vi "LEP_RV_ASW_BuildReportTab.vi"() -> ()   [LabVIEW 2011]
uses:
  resource/dialog/PreferencesDialog/optionsFrame_EventData1.ctl
panel:
  out "status display":string="Unknown"
  in  "eval mode?":bool
  in  "path to map file":path
  out "Unused":u32(colorbox)=16777215
  out "Other RAM":u32(colorbox)=12566942
  out "Heap RAM":u32(colorbox)=9328754
  out "RAM (kB)":cluster{dbl, dbl}(slide)={8.35820895522388, 30.80597014925373} scale=0.0..32.0
  out "Flash (kB)":dbl(slide)=29.611940298507463 scale=0.0..64.0
  out "Total Memory (%)":cluster{dbl, dbl, dbl, dbl}(slide)={31.343283582089555, 43.28358208955224, 61.194029850746276, 78.35820895522389} scale=0.0..100.0
  out "Flash Memory":u32(colorbox)=6654652
  out "Unavailable in Evaluation Mode":u32(colorbox)=1381653
  in  "page sync rendezvous":T1
  in  "error msg format string":string="There was a problem applying the options from the %s category. The error message is \"%s.\""
  in  "error in (no error)":errorcluster
  in  "Close Event":refnum<user-event>
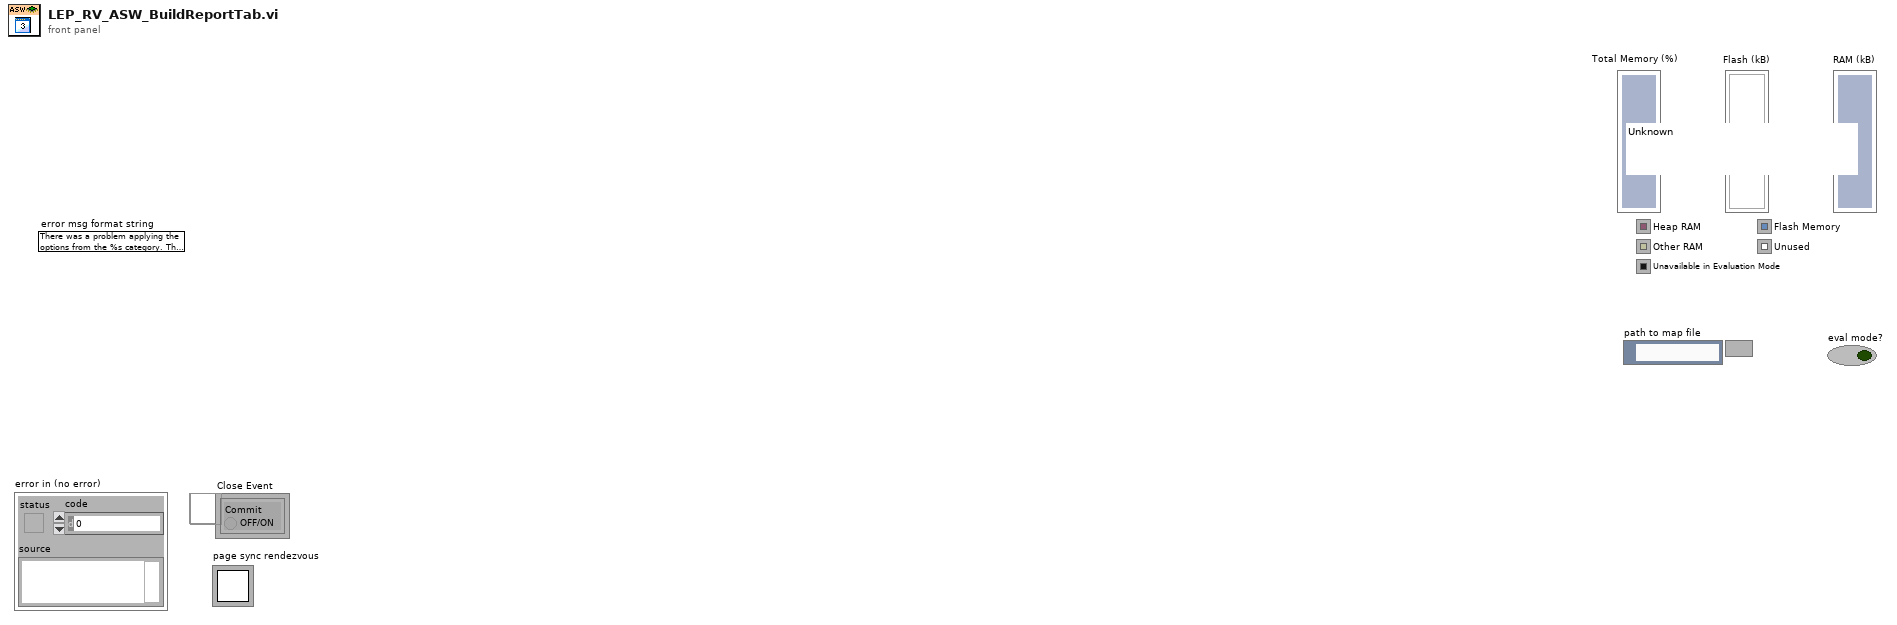
[diagram p1: front panel]
types:
  T1 = typedef "Rendezvous RefNum" = refnum<k1>
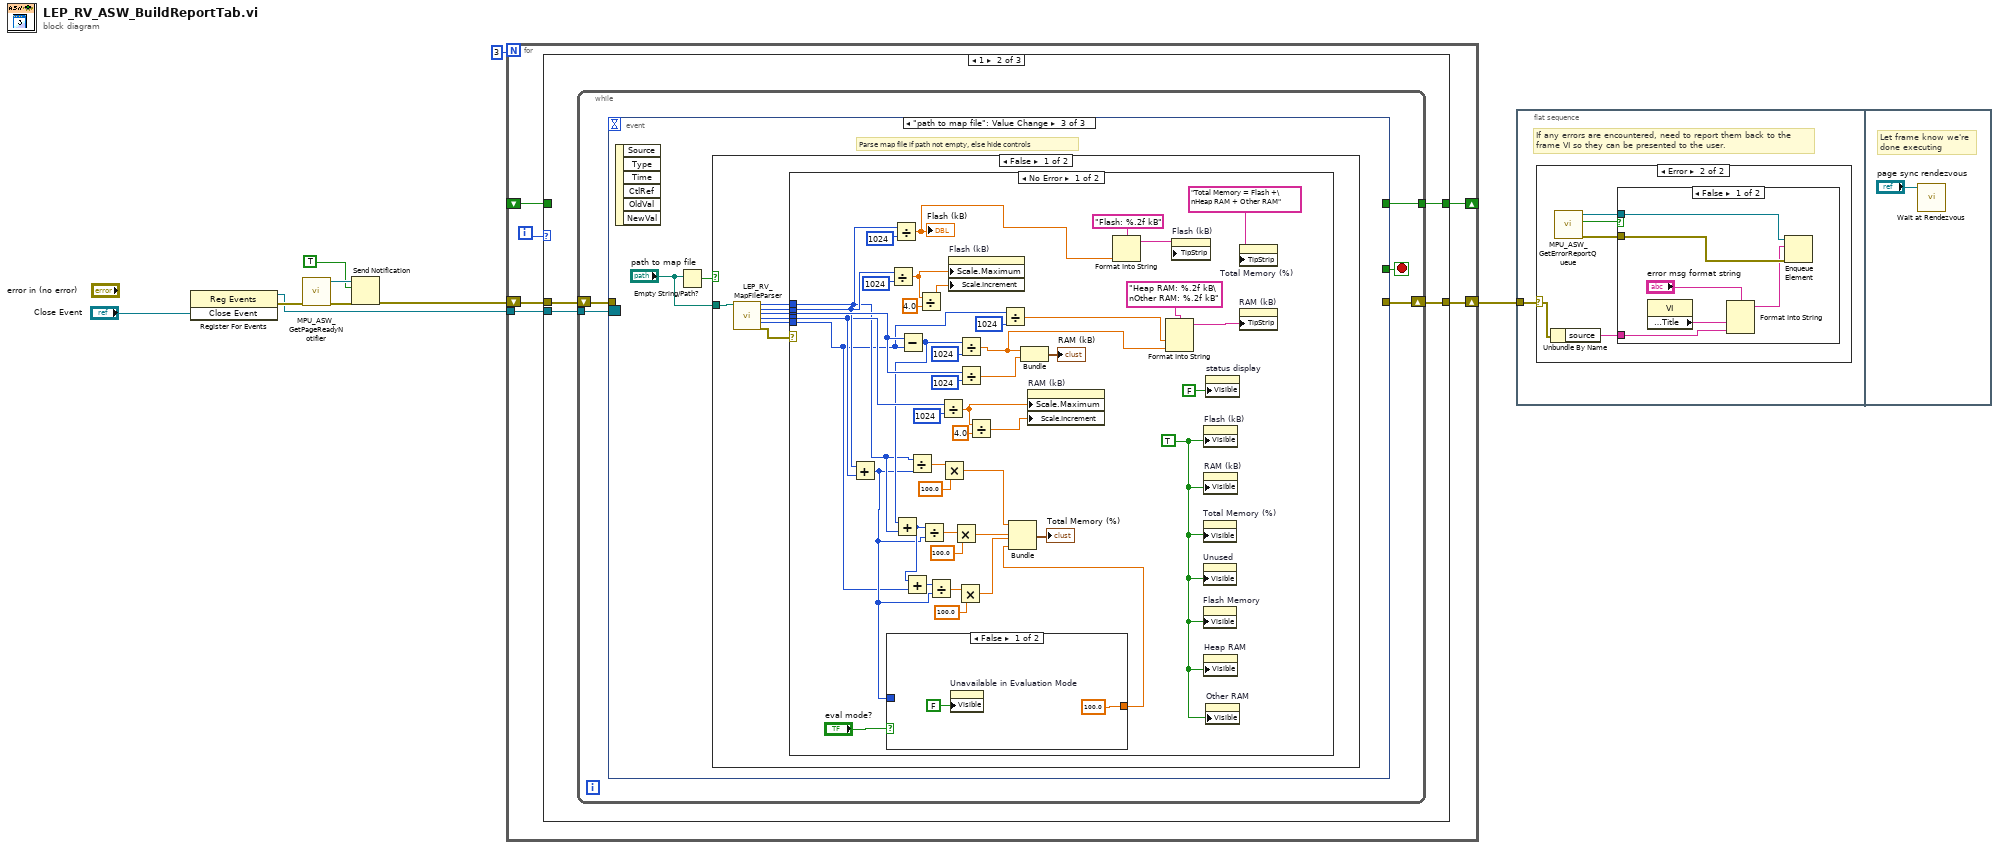
[diagram p0: block diagram]
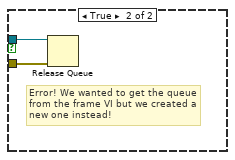
[diagram p3: hidden frame]
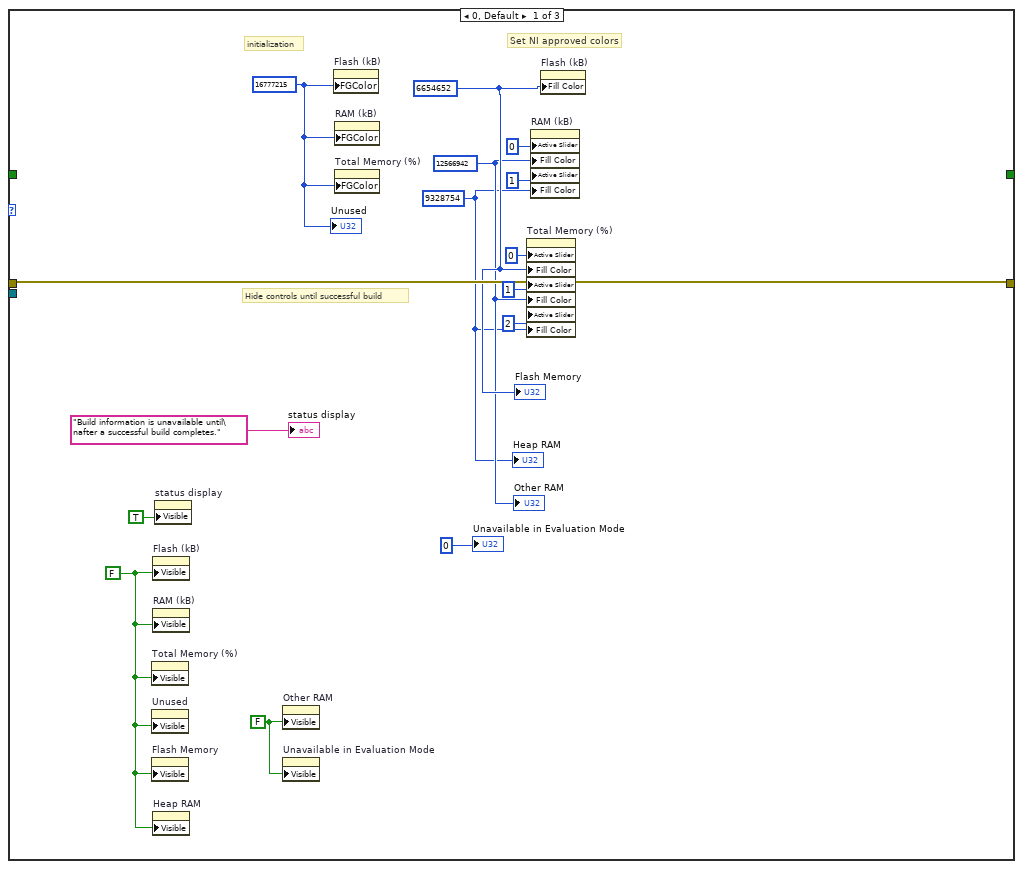
[diagram p4: hidden frame]
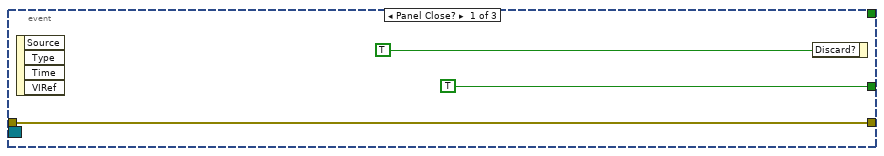
[diagram p5: hidden frame]
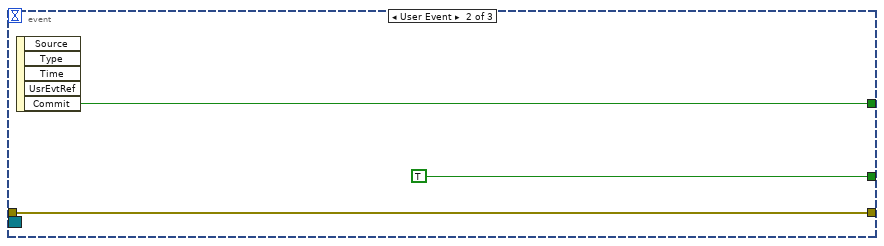
[diagram p6: hidden frame]
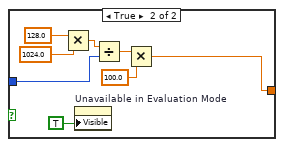
[diagram p7: hidden frame]
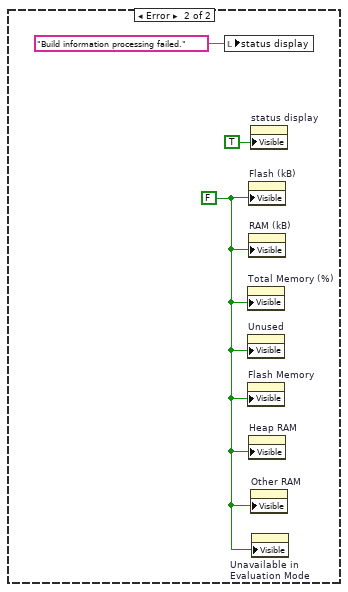
[diagram p8: hidden frame]
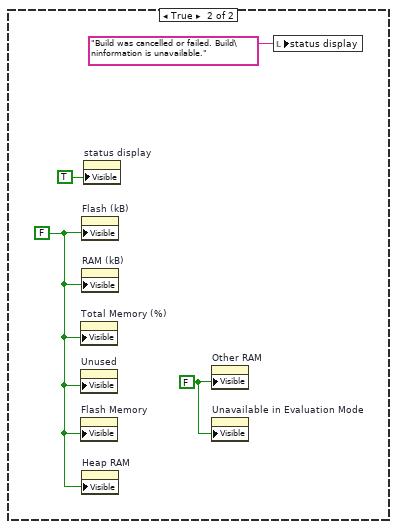
[diagram p9: hidden frame]
diagram:
  n1 = register-events("Close Event") -> (reference out=w4:refnum<event-registration>, error out=w6:errorcluster)  [unwired: 2 in]
  n2 = call "MPU_ASW_GetPageReadyNotifier.vi"("error in (no error)"=w6) -> ("error out"=w8:errorcluster, "notifier out"=w9:refnum<notifier>)  [unwired: 9 out]
  n3 = Send Notification(notification=TRUE, notifier=w9, error in (no error)=w8) -> (error out=w2:errorcluster)  [unwired: 1 out]
  n4 = for {
    N: 3 -> [_]
    shift-right: [w10] -> w3
    shift-left: w2 -> [w14]
    shift-right: [w13] -> _
    shift-left: _ -> [w12]
    tunnel: w4 -> [w11]
    i -> [w15]
    n5 = case shown="1" w15 {
      tunnel: w14 -> [w30 w34 w118]
      tunnel: [_ w31 _] -> w13
      tunnel: w12 -> [_ _ w119]
      tunnel: w11 -> [_ w33 _]
      tunnel: [w30 w32 w117] -> w10
      frame 0, Default {
        w19 = FALSE ("Visible")
        w18 = FALSE ("Visible")
        w20 = u32 9328754 ("Fill Style")
        w21 = u32 12566942 ("Fill Style")
        w24 = u32 6654652 ("Fill Style")
        w22 = u32 16777215 ("Fill Style")
        # "Hide controls until successful build"
        # "Set NI approved colors"
        # "initialization"
        n6 = property on="Total Memory (%)" class="Slide (strict)"("Visible"=w18) -> ()  [unwired: 2 in, 2 out]
        n7 = property on="Unused" class="ColBox"("Visible"=w18) -> ()  [unwired: 2 in, 2 out]
        n8 = property on="Flash Memory" class="ColBox"("Visible"=w18) -> ()  [unwired: 2 in, 2 out]
        n9 = property on="Flash (kB)" class="Slide (strict)"("Visible"=w18) -> ()  [unwired: 2 in, 2 out]
        n10 = property on="RAM (kB)" class="Slide (strict)"("Visible"=w18) -> ()  [unwired: 2 in, 2 out]
        n11 = property on="Heap RAM" class="ColBox"("Visible"=w18) -> ()  [unwired: 2 in, 2 out]
        n12 = property on="status display" class="Str"("Visible"=TRUE) -> ()  [unwired: 2 in, 2 out]
        n13 = property on="Other RAM" class="ColBox"("Visible"=w19) -> ()  [unwired: 2 in, 2 out]
        n14 = property on="Unavailable in Evaluation Mode" class="ColBox"("Visible"=w19) -> ()  [unwired: 2 in, 2 out]
        n15 = property on="Flash (kB)" class="Slide (strict)"("FGColor"=w22) -> ()  [unwired: 2 in, 2 out]
        n16 = property on="RAM (kB)" class="Slide (strict)"("FGColor"=w22) -> ()  [unwired: 2 in, 2 out]
        n17 = property on="Total Memory (%)" class="Slide (strict)"("FGColor"=w22) -> ()  [unwired: 2 in, 2 out]
        n18 = property on="Total Memory (%)" class="Slide (strict)"("Active Slider"=0, "Fill Color"=w24, "Active Slider"=1, "Fill Color"=w21, "Active Slider"=2, "Fill Color"=w20) -> ()  [unwired: 2 in, 2 out]
        n19 = property on="RAM (kB)" class="Slide (strict)"("Active Slider"=0, "Fill Color"=w21, "Active Slider"=1, "Fill Color"=w20) -> ()  [unwired: 2 in, 2 out]
        n20 = property on="Flash (kB)" class="Slide (strict)"("Fill Color"=w24) -> ()  [unwired: 2 in, 2 out]
        "Unavailable in Evaluation Mode" <- u32 0 ("Fill Style")
        "Flash Memory" <- w24
        "Heap RAM" <- w20
        "Other RAM" <- w21
        "Unused" <- w22
        "status display" <- "Build information is unavailable until\nafter a successful build completes." ("Text")
      }
      frame 1 {
        n21 = while {
          shift-right: [w38] -> w32
          shift-left: w34 -> [w39]
          tunnel: [w37] -> w31
          tunnel: w33 -> [w35]
          stop <- w36 stop-if-true
          n22 = event shown="[2] \"path to map file\": Value Change" {
            selector: w35 -> [_ _ _]
            dyn-events: _ -> [_ _ _]
            timeout: _ -> [_ _ _]
            tunnel: w39 -> [w41 w43 _]
            tunnel: [w41 w43 _] -> w38
            tunnel: [_ w45 _] -> w37
            tunnel: [TRUE TRUE _] -> w36
            event Panel Close? {
              n23 = event-data() -> ()  [unwired: 5 out]
              n24 = event-data("Discard?"=TRUE) -> ()  [unwired: 1 in, 1 out]
            }
            event User Event {
              n25 = event-data() -> ("Commit"=w45:bool)  [unwired: 5 out]
            }
            event "path to map file": Value Change {
              # "Parse map file if path not empty, else hide controls"
              n26 = event-data() -> ()  [unwired: 7 out]
              n27 = Empty String/Path?(string/path="path to map file") -> (empty?=w47:bool)
              n28 = case shown="False" w47 {
                tunnel: "path to map file" -> [w54 _]
                frame False {
                  n29 = call "LEP_RV_MapFileParser.vi"("map file"=w54) -> ("total used ROM"=w50:u32, "total available ROM"=w52:u32, "total used RAM"=w53:u32, "total available RAM"=w51:u32, "heap size"=w49:i32, "error out"=w48:errorcluster)  [unwired: 12 in, 1 out]
                  n30 = case shown="No Error" w48 {
                    tunnel: w53 -> [w87 _]
                    tunnel: w52 -> [w85 _]
                    tunnel: w51 -> [w84 _]
                    tunnel: w50 -> [w79 _]
                    tunnel: w49 -> [w58 _]
                    frame No Error {
                      w66 = TRUE ("Visible")
                      n31 = Add(x=w85, y=w84) -> (x+y=w68:u32)
                      n32 = case shown="False" "eval mode?" {
                        tunnel: [100.0 ("y") w103] -> w69
                        tunnel: w68 -> [_ w104]
                        frame False {
                          n33 = property on="Unavailable in Evaluation Mode" class="ColBox"("Visible"=FALSE) -> ()  [unwired: 2 in, 2 out]
                        }
                        frame True {
                          n34 = Multiply(x=128.0, y=1024.0) -> (x*y=w105:dbl)
                          n35 = property on="Unavailable in Evaluation Mode" class="ColBox"("Visible"=TRUE) -> ()  [unwired: 2 in, 2 out]
                          n36 = Divide(x=w105, y=w104) -> (x/y=w107:dbl)
                          n37 = Multiply(x=w107, y=100.0) -> (x*y=w103:dbl)
                        }
                      }
                      n38 = Divide(x=w85, y=u32 1024) -> (x/y=w96:dbl)
                      n39 = Divide(x=w79, y=u32 1024) -> (x/y=w64:dbl)
                      "Flash (kB)" <- w64
                      n40 = Subtract(x=w87, y=w58) -> (x-y=w80:u32)
                      n41 = Add(x=w80, y=w79) -> (x+y=w78:u32)
                      n42 = Add(x=w78, y=w58) -> (x+y=w77:u32)
                      n43 = Divide(x=w79, y=w68) -> (x/y=w83:dbl)
                      n44 = Divide(x=w96, y=4.0) -> (x/y=w95:dbl)
                      n45 = Divide(x=w78, y=w68) -> (x/y=w75:dbl)
                      n46 = Divide(x=w77, y=w68) -> (x/y=w73:dbl)
                      n47 = Divide(x=w84, y=u32 1024) -> (x/y=w88:dbl)
                      n48 = Multiply(x=w83, y=100.0) -> (x*y=w81:dbl)
                      n49 = property on="Flash (kB)" class="Slide (strict)"("Scale.Maximum"=w96, "Scale.Increment"=w95) -> ()  [unwired: 2 in, 2 out]
                      n50 = Multiply(x=w75, y=100.0) -> (x*y=w72:dbl)
                      n51 = Multiply(x=w73, y=100.0) -> (x*y=w71:dbl)
                      n52 = Divide(x=w80, y=u32 1024) -> (x/y=w55:dbl)
                      n53 = Divide(x=w87, y=u32 1024) -> (x/y=w56:dbl)
                      n54 = Divide(x=w88, y=4.0) -> (x/y=w89:dbl)
                      n55 = Divide(x=w58, y=u32 1024) -> (x/y=w57:dbl)
                      n56 = Bundle(w81, w72, w71, "y"=w69) -> (→"Total Memory (%)":cluster{dbl, dbl, dbl, "y":dbl})  [unwired: 1 in]
                      n57 = Bundle(w55, w56) -> (→"RAM (kB)":cluster{dbl, dbl})  [unwired: 1 in]
                      n58 = property on="RAM (kB)" class="Slide (strict)"("Scale.Maximum"=w88, "Scale.Increment"=w89) -> ()  [unwired: 2 in, 2 out]
                      n59 = Format Into String(format string="Flash: %.2f kB", w64) -> (resulting string=w62:string)  [unwired: 2 in, 1 out]
                      n60 = Format Into String(format string="Heap RAM: %.2f kB\nOther RAM: %.2f kB", w57, w55) -> (resulting string=w60:string)  [unwired: 2 in, 1 out]
                      n61 = property on="Flash (kB)" class="Slide (strict)"("TipStrip"=w62) -> ()  [unwired: 2 in, 2 out]
                      n62 = property on="Total Memory (%)" class="Slide (strict)"("Visible"=w66) -> ()  [unwired: 2 in, 2 out]
                      n63 = property on="Unused" class="ColBox"("Visible"=w66) -> ()  [unwired: 2 in, 2 out]
                      n64 = property on="Flash Memory" class="ColBox"("Visible"=w66) -> ()  [unwired: 2 in, 2 out]
                      n65 = property on="Flash (kB)" class="Slide (strict)"("Visible"=w66) -> ()  [unwired: 2 in, 2 out]
                      n66 = property on="RAM (kB)" class="Slide (strict)"("Visible"=w66) -> ()  [unwired: 2 in, 2 out]
                      n67 = property on="Heap RAM" class="ColBox"("Visible"=w66) -> ()  [unwired: 2 in, 2 out]
                      n68 = property on="status display" class="Str"("Visible"=FALSE) -> ()  [unwired: 2 in, 2 out]
                      n69 = property on="Other RAM" class="ColBox"("Visible"=w66) -> ()  [unwired: 2 in, 2 out]
                      n70 = property on="Total Memory (%)" class="Slide (strict)"("TipStrip"="Total Memory = Flash +\nHeap RAM + Other RAM" ("format string")) -> ()  [unwired: 2 in, 2 out]
                      n71 = property on="RAM (kB)" class="Slide (strict)"("TipStrip"=w60) -> ()  [unwired: 2 in, 2 out]
                    }
                    frame Error {
                      w112 = FALSE ("Visible")
                      n72 = local write "status display"("Build information processing failed." ("status display")) -> ()
                      n73 = property on="Total Memory (%)" class="Slide (strict)"("Visible"=w112) -> ()  [unwired: 2 in, 2 out]
                      n74 = property on="Unused" class="ColBox"("Visible"=w112) -> ()  [unwired: 2 in, 2 out]
                      n75 = property on="Flash Memory" class="ColBox"("Visible"=w112) -> ()  [unwired: 2 in, 2 out]
                      n76 = property on="Flash (kB)" class="Slide (strict)"("Visible"=w112) -> ()  [unwired: 2 in, 2 out]
                      n77 = property on="RAM (kB)" class="Slide (strict)"("Visible"=w112) -> ()  [unwired: 2 in, 2 out]
                      n78 = property on="Heap RAM" class="ColBox"("Visible"=w112) -> ()  [unwired: 2 in, 2 out]
                      n79 = property on="status display" class="Str"("Visible"=TRUE) -> ()  [unwired: 2 in, 2 out]
                      n80 = property on="Other RAM" class="ColBox"("Visible"=w112) -> ()  [unwired: 2 in, 2 out]
                      n81 = property on="Unavailable in Evaluation Mode" class="ColBox"("Visible"=w112) -> ()  [unwired: 2 in, 2 out]
                    }
                  }
                }
                frame True {
                  w116 = FALSE ("Visible")
                  w115 = FALSE ("Visible")
                  n82 = property on="Total Memory (%)" class="Slide (strict)"("Visible"=w115) -> ()  [unwired: 2 in, 2 out]
                  n83 = property on="Unused" class="ColBox"("Visible"=w115) -> ()  [unwired: 2 in, 2 out]
                  n84 = property on="Flash Memory" class="ColBox"("Visible"=w115) -> ()  [unwired: 2 in, 2 out]
                  n85 = property on="Flash (kB)" class="Slide (strict)"("Visible"=w115) -> ()  [unwired: 2 in, 2 out]
                  n86 = property on="RAM (kB)" class="Slide (strict)"("Visible"=w115) -> ()  [unwired: 2 in, 2 out]
                  n87 = property on="Heap RAM" class="ColBox"("Visible"=w115) -> ()  [unwired: 2 in, 2 out]
                  n88 = property on="status display" class="Str"("Visible"=TRUE) -> ()  [unwired: 2 in, 2 out]
                  n89 = property on="Other RAM" class="ColBox"("Visible"=w116) -> ()  [unwired: 2 in, 2 out]
                  n90 = property on="Unavailable in Evaluation Mode" class="ColBox"("Visible"=w116) -> ()  [unwired: 2 in, 2 out]
                  n91 = local write "status display"("Build was cancelled or failed. Build\ninformation is unavailable." ("status display")) -> ()
                }
              }
            }
          }
        }
      }
      frame 2 {
        n92 = case shown="True" w119 {
          tunnel: w118 -> [w120 w121]
          tunnel: [w120 w121] -> w117
          frame False {
          }
          frame True {
          }
        }
      }
    }
  }
  n93 = flat-sequence {
    tunnel: w3 -> [w122]
    frame #0 {
      # "If any errors are encountered, need to report them back to the \nframe VI so they can be presented to the user."
      n94 = case shown="Error" w122 {
        selector: w122 -> [_ w124]
        frame No Error {
        }
        frame Error {
          n95 = Unbundle By Name(w124) -> ("source"=w123:string)
          n96 = call "MPU_ASW_GetErrorReportQueue.vi"() -> ("error out"=w125:errorcluster, "created new?"=w127:bool, "queue out"=w126:refnum<queue>)  [unwired: 9 out]
          n97 = case shown="False" w127 {
            tunnel: w126 -> [w133 w135]
            tunnel: w125 -> [w132 w134]
            tunnel: w123 -> [w129 _]
            frame False {
              n98 = property class="VI"() -> ("Front Panel.Title"=w130:string)  [unwired: 2 in, 2 out]
              n99 = Format Into String(format string="error msg format string", w130, w129) -> (resulting string=w128:string)  [unwired: 2 in, 1 out]
              n100 = Enqueue Element(queue=w133, element=w128, error in (no error)=w132) -> ()  [unwired: 4 out]
            }
            frame True {
              # "Error! We wanted to get the queue\nfrom the frame VI but we created a\nnew one instead!"
              n101 = Release Queue(queue=w135, error in (no error)=w134) -> ()  [unwired: 4 out]
            }
          }
        }
      }
    }
    frame #1 {
      # "Let frame know we're \ndone executing"
      n102 = call <vilib>:"Wait at Rendezvous.vi"("rendezvous"="page sync rendezvous") -> ()  [unwired: 2 in, 5 out]
    }
  }
